vi "BlobDrawer.vi"(2 "BlobData In":dbl[][](array[numeric]), 3 "Image In":T2) -> (0 "BlobData":T1(array[cluster]), 1 "Image Out":T2)   [LabVIEW 2011]
uses:
  <vilib>/vision/Image Controls.llb/IMAQ Image.ctl
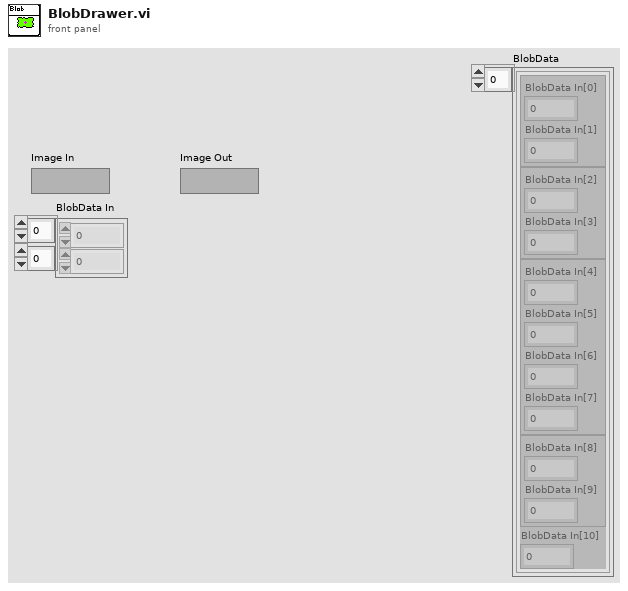
[diagram p1: front panel]
types:
  T1 = cluster{cluster{"BlobData In[0]":dbl, "BlobData In[1]":dbl}, cluster{"BlobData In[2]":dbl, "BlobData In[3]":dbl}, cluster{"BlobData In[4]":dbl, "BlobData In[5]":dbl, "BlobData In[6]":dbl, "BlobData In[7]":dbl}, cluster{"BlobData In[8]":dbl, "BlobData In[9]":dbl}, "BlobData In[10]":dbl}[]
  T2 = typedef "IMAQ Image.ctl" = refnum<image>
  T3 = cluster{"BlobData In[0]":dbl, "BlobData In[1]":dbl, "BlobData In[2]":dbl, "BlobData In[3]":dbl, "BlobData In[4]":dbl, "BlobData In[5]":dbl, "BlobData In[6]":dbl, "BlobData In[7]":dbl, "BlobData In[8]":dbl, "BlobData In[9]":dbl, "BlobData In[10]":dbl}
  T4 = cluster{"BlobData In[0]":dbl, "BlobData In[1]":dbl}
  T5 = cluster{"BlobData In[2]":dbl, "BlobData In[3]":dbl}
  T6 = cluster{"BlobData In[4]":dbl, "BlobData In[5]":dbl, "BlobData In[6]":dbl, "BlobData In[7]":dbl}
  T7 = cluster{"BlobData In[8]":dbl, "BlobData In[9]":dbl}
  T8 = cluster{cluster{"BlobData In[0]":dbl, "BlobData In[1]":dbl}, cluster{"BlobData In[2]":dbl, "BlobData In[3]":dbl}, cluster{"BlobData In[4]":dbl, "BlobData In[5]":dbl, "BlobData In[6]":dbl, "BlobData In[7]":dbl}, cluster{"BlobData In[8]":dbl, "BlobData In[9]":dbl}, "BlobData In[10]":dbl}
  T9 = cluster{"BlobData In[0]":dbl, "BlobData In[1]":dbl, "BlobData In[0]":dbl, "BlobData In[1]":dbl}
  T10 = cluster{"BlobData In[2]":dbl, "BlobData In[3]":dbl, "BlobData In[2]":dbl, "BlobData In[3]":dbl}
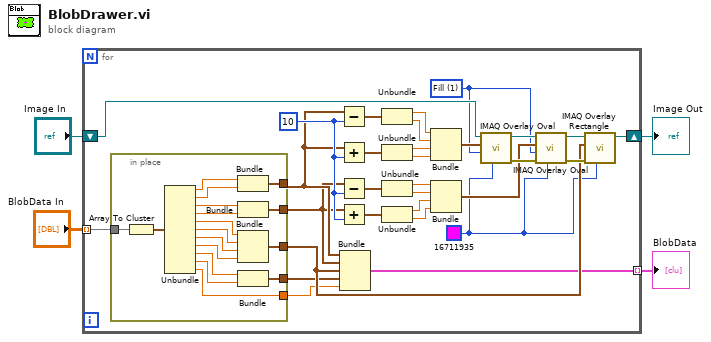
[diagram p0: block diagram]
diagram:
  n1 = for {
    tunnel: "BlobData In" -> [w34] mode=indexing
    shift-right: [w12] -> w2
    shift-left: "Image In" -> [w33]
    tunnel: [w6] -> w1 mode=indexing
    w5 = u32 16711935 ("Color")
    w15 = u32 1 items=["Frame", "Fill"] ("Drawing Mode (Frame)")
    w32 = 10
    n2 = in-place {
      in-place-border: w34 -> [w51]
      in-place-border: [w39] -> w11
      in-place-border: [w38] -> w10
      in-place-border: [w37] -> w9
      in-place-border: [w36] -> w8
      in-place-border: [w35] -> w7
      n3 = Array To Cluster(array=w51) -> (cluster=w50:T3)
      n4 = Unbundle(w50) -> ("BlobData In[0]"=w49:dbl, "BlobData In[1]"=w48:dbl, "BlobData In[2]"=w47:dbl, "BlobData In[3]"=w46:dbl, "BlobData In[4]"=w45:dbl, "BlobData In[5]"=w44:dbl, "BlobData In[6]"=w43:dbl, "BlobData In[7]"=w42:dbl, "BlobData In[8]"=w41:dbl, "BlobData In[9]"=w40:dbl, "BlobData In[10]"=w35:dbl)
      n5 = Bundle("BlobData In[0]"=w49, "BlobData In[1]"=w48) -> (w39:T4)  [unwired: 1 in]
      n6 = Bundle("BlobData In[2]"=w47, "BlobData In[3]"=w46) -> (w38:T5)  [unwired: 1 in]
      n7 = Bundle("BlobData In[4]"=w45, "BlobData In[5]"=w44, "BlobData In[6]"=w43, "BlobData In[7]"=w42) -> (w37:T6)  [unwired: 1 in]
      n8 = Bundle("BlobData In[8]"=w41, "BlobData In[9]"=w40) -> (w36:T7)  [unwired: 1 in]
    }
    n9 = Subtract(x=w11, y=w32) -> (x-y=w31:T4)
    n10 = Add(x=w11, y=w32) -> (x+y=w30:T4)
    n11 = Subtract(x=w10, y=w32) -> (x-y=w29:T5)
    n12 = Add(x=w10, y=w32) -> (x+y=w28:T5)
    n13 = Bundle(w11, w10, w9, w8, "BlobData In[10]"=w7) -> (w6:T8)  [unwired: 1 in]
    n14 = Unbundle(w31) -> ("BlobData In[0]"=w27:dbl, "BlobData In[1]"=w24:dbl)
    n15 = Unbundle(w30) -> ("BlobData In[0]"=w25:dbl, "BlobData In[1]"=w26:dbl)
    n16 = Unbundle(w29) -> ("BlobData In[2]"=w23:dbl, "BlobData In[3]"=w22:dbl)
    n17 = Unbundle(w28) -> ("BlobData In[2]"=w21:dbl, "BlobData In[3]"=w20:dbl)
    n18 = Bundle("BlobData In[0]"=w27, "BlobData In[1]"=w24, "BlobData In[0]"=w25, "BlobData In[1]"=w26) -> (w17:T9)  [unwired: 1 in]
    n19 = Bundle("BlobData In[2]"=w23, "BlobData In[3]"=w22, "BlobData In[2]"=w21, "BlobData In[3]"=w20) -> (w16:T10)  [unwired: 1 in]
    n20 = call "IMAQ Overlay Oval"("Color"=w5, "Drawing Mode (Frame)"=w15, "Bounding Rectangle"=w17, "Image"=w33) -> ("error out"=w19:errorcluster, "Image Out"=w18:T2)  [unwired: 6 in]
    n21 = call "IMAQ Overlay Oval"("Color"=w5, "error in (no error)"=w19, "Drawing Mode (Frame)"=w15, "Bounding Rectangle"=w16, "Image"=w18) -> ("error out"=w14:errorcluster, "Image Out"=w13:T2)  [unwired: 5 in]
    n22 = call "IMAQ Overlay Rectangle"("Color"=w5, "error in (no error)"=w14, "Rectangle"=w9, "Image"=w13) -> ("Image Out"=w12:T2)  [unwired: 6 in, 1 out]
  }
  "Image Out" <- w2
  "BlobData" <- w1
